vi "Add Target.vi"(7 "Overwrite Existing?":bool=TRUE, 8 "error in (no error)":errorcluster, 9 "Settings":T2={"Name"="Controller", "Target Type"="Windows", "IPAddress"="localhost", "PrimaryControlLoopProcessor"=-2, "DataProcessingLoopProcessor"=-2, "DataProcessingLoopDecimation"=1, "DAQDigitalLinesDecimation"=1, "MaximumStreamedChannels"=512, "ExecutionMode"=0, "FilterDAQErrors"=FALSE, "FilterWatchdogErrors"=FALSE, "FPGAScanInterfaceMode"=0, "TargetRate"=100.0} {"FPGAScanInterfaceMode" items=["Use Current", "FPGA Mode", "Scan Mode"]; "ExecutionMode" items=["Parallel", "LowLatency"]}, 11 "SysDef Ref":T4) -> (0 "error out":errorcluster, 2 "Target Node Paths":T1, 3 "SysDef Ref Out":T4)   [LabVIEW 2019, in "Simple SysDef API.lvlib"]
uses:
  <userlib>/SimpleSysDef/Simple SysDef API.lvlib
  <userlib>/SimpleSysDef/_SubVIs/System Definition Reference.ctl
  NationalInstruments.VeriStand.SystemDefinitionAPI
  <userlib>/SimpleSysDef/_SubVIs/Add Target_Settings.ctl
  <userlib>/SimpleSysDef/_SubVIs/Add Target_Types.ctl
  <userlib>/SimpleSysDef/_SubVIs/Target Node Paths.ctl
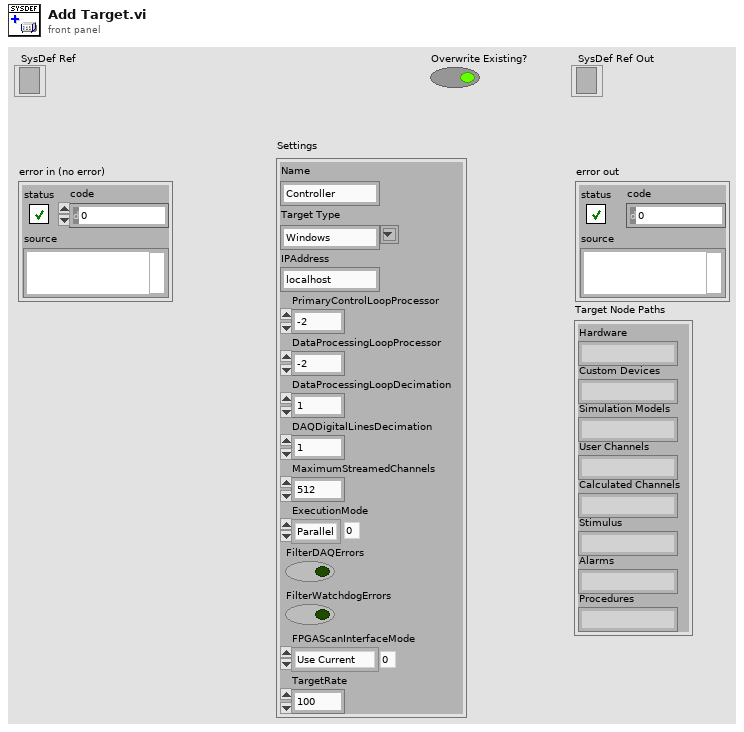
[diagram p1: front panel]
types:
  T1 = typedef "Simple SysDef API.lvlib/Target Node Paths.ctl" = cluster{"Hardware":string, "Custom Devices":string, "Simulation Models":string, "User Channels":string, "Calculated Channels":string, "Stimulus":string, "Alarms":string, "Procedures":string}
  T2 = typedef "Simple SysDef API.lvlib/Add Target_Settings.ctl" = cluster{"Name":string, "Target Type":T3, "IPAddress":string, "PrimaryControlLoopProcessor":i32, "DataProcessingLoopProcessor":i32, "DataProcessingLoopDecimation":i32, "DAQDigitalLinesDecimation":u32, "MaximumStreamedChannels":i32, "ExecutionMode":i32, "FilterDAQErrors":bool, "FilterWatchdogErrors":bool, "FPGAScanInterfaceMode":u16, "TargetRate":dbl}
  T3 = typedef "Simple SysDef API.lvlib/Add Target_Types.ctl" = string
  T4 = typedef "Simple SysDef API.lvlib/System Definition Reference.ctl" = refnum<k24>
  T5 = cluster{"[0]":string, "[1]":string, "[2]":string, "[3]":string, "[4]":string, "[5]":string, "[6]":string, "[7]":string}
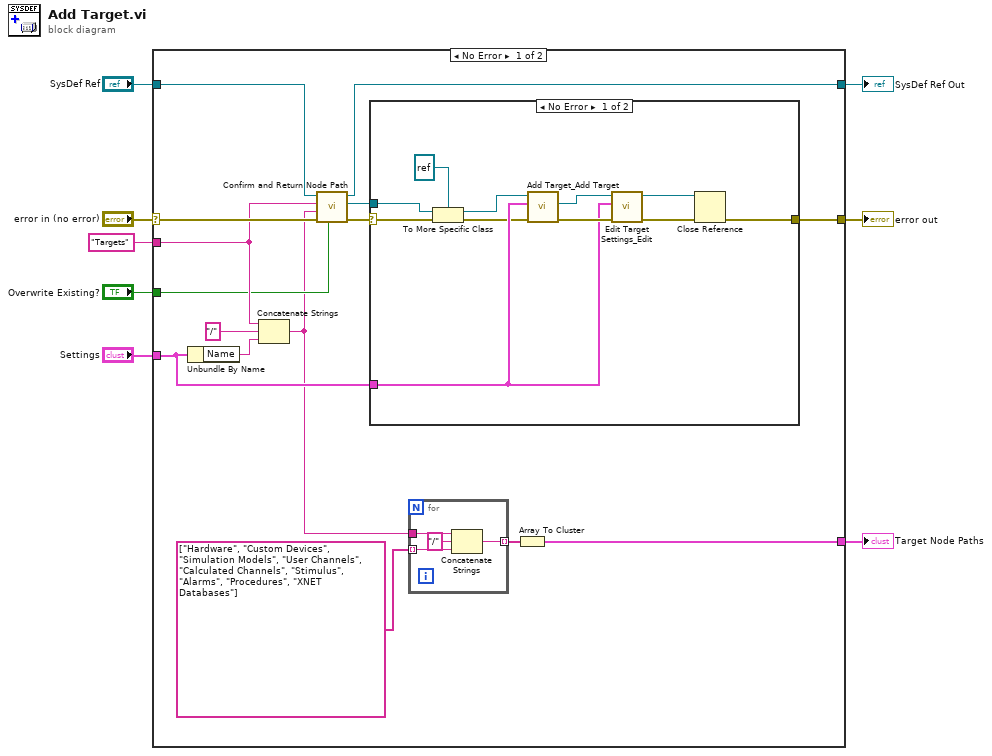
[diagram p0: block diagram]
diagram:
  n1 = case shown="No Error" "error in (no error)" {
    selector: "error in (no error)" -> [w23 w41]
    tunnel: [w18 w41] -> w3
    tunnel: "SysDef Ref" -> [w22 w40]
    tunnel: [w21 w40] -> w2
    tunnel: "Targets" ("System Definition Node Path") -> [w15 _]
    tunnel: "Overwrite Existing?" -> [w14 _]
    tunnel: "Settings" -> [w13 _]
    tunnel: [w9 _] -> w1
    frame No Error {
      n2 = Unbundle By Name(w13) -> ("Name"=w19:string)
      n3 = Concatenate Strings(w15, "/" ("string"), w19) -> (w12:string)
      n4 = call <userlib>:"Confirm and Return Node Path.vi"("Overwrite Existing?"=w14, "error in (no error)"=w23, "New Node Path"=w12, "Base Node Path"=w15, "SysDef Ref"=w22) -> ("error out"=w16:errorcluster, "Node Ref"=w17:refnum<k24>, "SysDef Ref Out"=w21:T4)  [unwired: 4 in]
      n5 = case shown="No Error" w16 {
        selector: w16 -> [w37 w39]
        tunnel: [w31 w39] -> w18
        tunnel: w17 -> [w38 _]
        tunnel: w13 -> [w35 _]
        frame No Error {
          n6 = To More Specific Class(target class=refnum<k24> refnum ("Node Ref"), reference=w38, error in=w37) -> (specific class reference=w29:refnum<k24>, error out=w33:errorcluster)
          n7 = call <userlib>:"Add Target_Add Target.vi"("error in (no error)"=w33, "Settings"=w35, "Targets Ref"=w29) -> ("error out"=w36:errorcluster, "Target Reference"=w28:refnum<k24>)  [unwired: 7 in]
          n8 = call <userlib>:"Edit Target Settings_Edit.vi"("error in (no error)"=w36, "Settings"=w35, "Target Ref"=w28) -> ("error out"=w32:errorcluster, "Target Ref Out"=w30:refnum<k24>)  [unwired: 7 in]
          n9 = Close Reference(reference=w30, error in (no error)=w32) -> (error out=w31:errorcluster)
        }
        frame Error {
        }
      }
      n10 = for {
        tunnel: w12 -> [w27]
        tunnel: string[] ["Hardware", "Custom Devices", "Simulation Models", "User Channels", "Calculated Channels", "Stimulus", "Alarms", "Procedures", "XNET Databases"] -> [w25] mode=indexing
        tunnel: [w24] -> w10 mode=indexing
        n11 = Concatenate Strings(w27, "/" ("string"), w25) -> (w24:string)
      }
      n12 = Array To Cluster(array=w10) -> (cluster=w9:T5)
    }
    frame Error {
    }
  }
  "SysDef Ref Out" <- w2
  "error out" <- w3
  "Target Node Paths" <- w1
